vi "Open Instrument.vi"(8 "error in (no error)":errorcluster, 11 "instrument.PPMS in":refnum<class "instrument.PPMS3.lvclass">) -> (0 "error out":errorcluster, 3 "instrument.PPMS out":refnum<class "instrument.PPMS3.lvclass">)   [LabVIEW 2016, in "instrument.PPMS3.lvclass"]
uses:
  instrument.PPMS3.lvclass
  C:/Program Files (x86)/National Instruments/LabVIEW 2016/user.lib/LevyLab/Levylab Instruments/SMOs/Instrument/Instrument.lvclass
  <userlib>/LevyLab/Levylab Instruments/SMOs/Instrument/Instrument.lvclass/Instrument.ctl
  instrument.PPMS3.lvclass/instrument.PPMS3.ctl
  <userlib>/LevyLab/Levylab Instruments/SMOs/Instrument/Instrument.lvclass
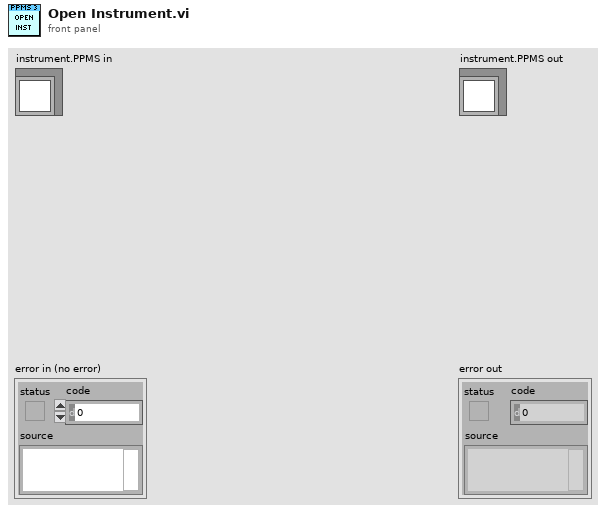
[diagram p1: front panel]
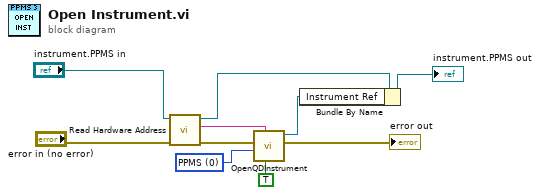
[diagram p0: block diagram]
diagram:
  w9 = 0 items=["PPMS", "VersaLab", "DynaCool", "SVSM"] ("Instrument\nType")
  n1 = call <userlib>:"Read Hardware Address.vi"("error in (no error)"="error in (no error)", "Instrument in"="instrument.PPMS in") -> ("error out"=w6:errorcluster, "Address"=w5:string, "Instrument out"=w3:refnum<class "instrument.PPMS3.lvclass">)  [unwired: 7 in]
  n2 = call "OpenQDInstrument.vi"("Remote"=TRUE, "IP Address"=w5, "Instrument Type"=w9, "error in (no error)"=w6) -> ("error out"=→"error out":errorcluster, "Instrument Ref"=w1:refnum<k24>)  [unwired: 4 in]
  n3 = Bundle By Name(cluster=w3, "Instrument Ref"=w1) -> (→"instrument.PPMS out":refnum<class "instrument.PPMS3.lvclass">)
